vi "Lock-in Globles Multiple Inputs and Outputs used with FGV.vi"() -> ()   [LabVIEW 2013]
panel:
  out "Reset Lockin":bool
  out "timestamp":timestamp
  in  "Multiplication factor":dbl=1.0
  out "Stop Read current vs T":bool
  out "Stop Lockin":bool
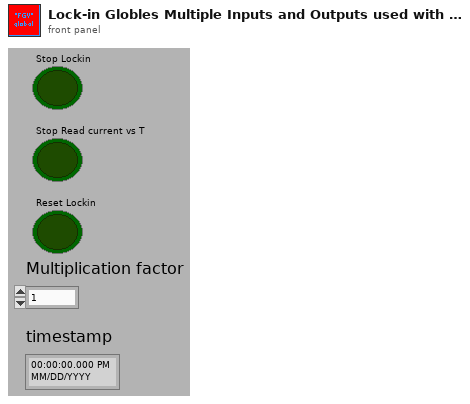
[diagram p1: front panel]
diagram:
